vi "EXCLUDE_COLOR.vi"() -> (2 "Color Box":u32(colorbox)=13816530)   [LabVIEW 2020, in "AbstractMultiColumnListBoxAdapter.lvclass"]
uses:
  AbstractMultiColumnListBoxAdapter.lvclass
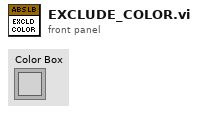
[diagram p1: front panel]
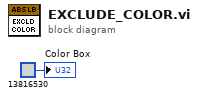
[diagram p0: block diagram]
diagram:
  "Color Box" <- u32 13816530
